vi "AddRefsToObject.vi"(8 "error in (no error)":errorcluster, 9 "Controls[]":refnum<vi>[](array[refnum]), 10 "VI Refnum":refnum<vi>, 11 "FolloWin in":refnum<class "FolloWin.lvclass">) -> (0 "error out":errorcluster, 3 "FolloWin out":refnum<class "FolloWin.lvclass">)   [LabVIEW 2023, in "FolloWin.lvclass"]
doc: "This VI extracts the references of the controls in FolloWin.vi and adds them to the object."
uses:
  FolloWin.lvclass
  FolloWin.lvclass/FolloWin.ctl
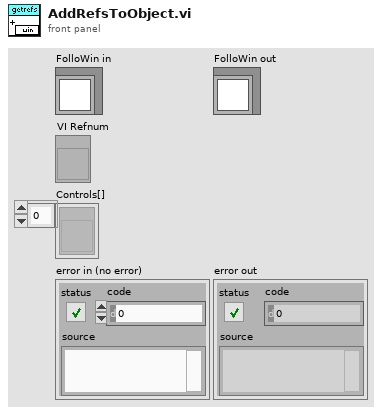
[diagram p1: front panel]
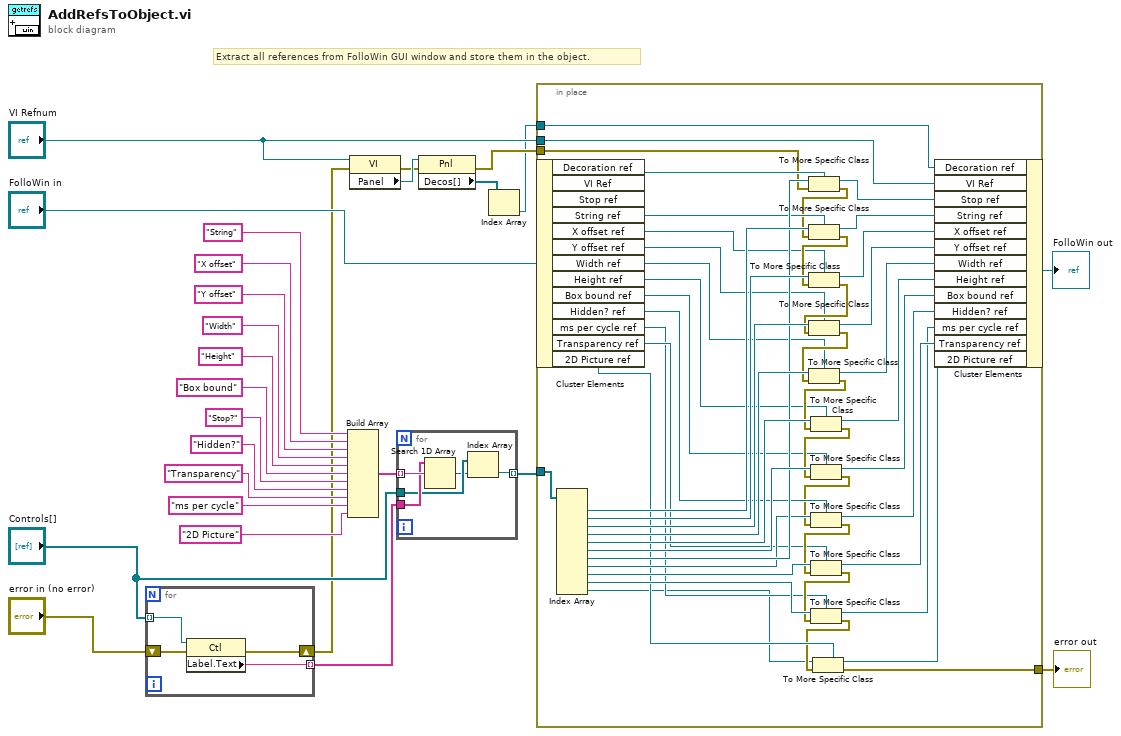
[diagram p0: block diagram]
diagram:
  # "Extract all references from FolloWin GUI window and store them in the object."
  n1 = for {
    tunnel: "Controls[]" -> [w30] mode=indexing
    tunnel: [w29] -> w14 mode=indexing
    shift-right: [w27] -> w3
    shift-left: "error in (no error)" -> [w28]
    n2 = property on="Property Node" class="Ctl"(reference=w30, error in=w28) -> (error out=w27:errorcluster, "Label.Text"=w29:string)  [unwired: 1 out]
  }
  n3 = Build Array("String", "X offset" ("element"), "Y offset" ("element"), "Width" ("element"), "Height" ("element"), "Box bound", "Stop?", "Hidden?", "Transparency", "ms per cycle", "2D Picture") -> (w15:string[])
  n4 = property on="Property Node" class="VI"(reference="VI Refnum", error in=w3) -> (error out=w5:errorcluster, "Panel"=w7:refnum<vi>)  [unwired: 1 out]
  n5 = for {
    tunnel: w15 -> [w35] mode=indexing
    tunnel: w14 -> [w34]
    tunnel: "Controls[]" -> [w33]
    tunnel: [w31] -> w12 mode=indexing
    n6 = Search 1D Array(1D array=w34, element=w35) -> (index of element=w32:i32)  [unwired: 1 in]
    n7 = Index Array(array=w33, index=w32) -> (element=w31:refnum<vi>)
  }
  n8 = property on="Property Node" class="Pnl"(reference=w7, error in=w5) -> (error out=w2:errorcluster, "Decos[]"=w6:refnum<vi>[])  [unwired: 1 out]
  n9 = Index Array(array=w6) -> (element=w1:refnum<vi>)  [unwired: 1 in]
  n10 = in-place "In Place Element Structure" {
    in-place-border: w12 -> [w83]
    in-place-border: [w39] -> w11
    in-place-border: w2 -> [w44]
    in-place-border: "VI Refnum" -> [w42]
    in-place-border: w1 -> [w36]
    n11 = in-place-cluster #1("FolloWin in") -> ("Stop ref"=w59:refnum<vi>, "String ref"=w65:refnum<vi>, "X offset ref"=w64:refnum<vi>, "Y offset ref"=w63:refnum<vi>, "Width ref"=w62:refnum<vi>, "Height ref"=w61:refnum<vi>, "Box bound ref"=w60:refnum<vi>, "Hidden? ref"=w58:refnum<vi>, "ms per cycle ref"=w56:refnum<vi>, "Transparency ref"=w57:refnum<vi>, "2D Picture ref"=w41:refnum<vi>)  [unwired: 2 out]
    n12 = Index Array(array=w83) -> (element #1=w82:refnum<vi>, element #2=w81:refnum<vi>, element #3=w80:refnum<vi>, element #4=w79:refnum<vi>, element #5=w78:refnum<vi>, element #6=w77:refnum<vi>, element #7=w76:refnum<vi>, element #8=w75:refnum<vi>, element #9=w74:refnum<vi>, element #10=w73:refnum<vi>, element #11=w37:refnum<vi>)  [unwired: 11 in]
    n13 = To More Specific Class(target class=w59, reference=w76, error in=w44) -> (specific class reference=w49:refnum<vi>, error out=w45:errorcluster)
    n14 = To More Specific Class(target class=w65, reference=w82, error in=w45) -> (specific class reference=w55:refnum<vi>, error out=w72:errorcluster)
    n15 = To More Specific Class(target class=w64, reference=w81, error in=w72) -> (specific class reference=w54:refnum<vi>, error out=w71:errorcluster)
    n16 = To More Specific Class(target class=w63, reference=w80, error in=w71) -> (specific class reference=w53:refnum<vi>, error out=w70:errorcluster)
    n17 = To More Specific Class(target class=w62, reference=w79, error in=w70) -> (specific class reference=w52:refnum<vi>, error out=w69:errorcluster)
    n18 = To More Specific Class(target class=w61, reference=w78, error in=w69) -> (specific class reference=w51:refnum<vi>, error out=w68:errorcluster)
    n19 = To More Specific Class(target class=w60, reference=w77, error in=w68) -> (specific class reference=w50:refnum<vi>, error out=w43:errorcluster)
    n20 = To More Specific Class(target class=w58, reference=w75, error in=w43) -> (specific class reference=w48:refnum<vi>, error out=w67:errorcluster)
    n21 = To More Specific Class(target class=w57, reference=w74, error in=w67) -> (specific class reference=w47:refnum<vi>, error out=w66:errorcluster)
    n22 = To More Specific Class(target class=w56, reference=w73, error in=w66) -> (specific class reference=w46:refnum<vi>, error out=w38:errorcluster)
    n23 = To More Specific Class(target class=w41, reference=w37, error in=w38) -> (specific class reference=w40:refnum<vi>, error out=w39:errorcluster)
    n24 = in-place-cluster #1("Decoration ref"=w36, "VI Ref"=w42, "Stop ref"=w49, "String ref"=w55, "X offset ref"=w54, "Y offset ref"=w53, "Width ref"=w52, "Height ref"=w51, "Box bound ref"=w50, "Hidden? ref"=w48, "ms per cycle ref"=w46, "Transparency ref"=w47, "2D Picture ref"=w40) -> (→"FolloWin out":refnum<class "FolloWin.lvclass">)
  }
  "error out" <- w11
